vi "Last element.vi"(11 "Circuit cluster":T1) -> (3 "Last element?":bool)   [LabVIEW 2016]
uses:
  TypeDefs/Circuit Cluster.ctl
  Classes/GateAbst/GateAbst.lvclass
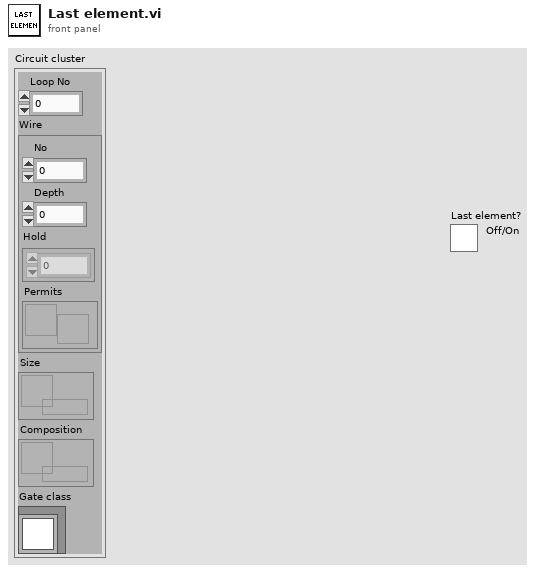
[diagram p1: front panel]
types:
  T1 = typedef "Circuit Cluster.ctl" = cluster{"Loop No":i32, "Wire":cluster{"No":i32, "Depth":i32, "Hold":i32[][], "Permits":refnum<notifier>}, "Size":refnum<queue>, "Composition":refnum<queue>, "Gate class":refnum<class "GateAbst.lvclass">}
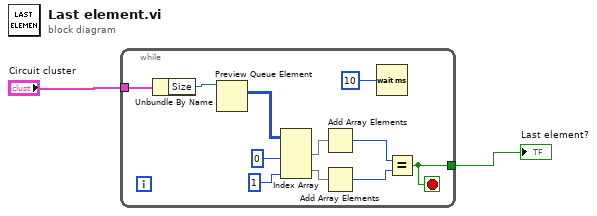
[diagram p0: block diagram]
diagram:
  n1 = while {
    tunnel: "Circuit cluster" -> [w12]
    tunnel: [w3] -> w2
    stop <- w3 stop-if-true
    n2 = Unbundle By Name(w12) -> ("Size"=w11:refnum<queue>)
    n3 = Preview Queue Element(queue=w11) -> (element=w13:i32[][])  [unwired: 2 in, 3 out]
    n4 = Index Array(array=w13, index (col) #1=0 ("disabled index (col)"), index (col) #2=1 ("index (col)")) -> (element #1=w7:i32[], element #2=w6:i32[])  [unwired: 2 in]
    n5 = Add Array Elements(numeric array=w7) -> (sum=w5:i32)
    n6 = Add Array Elements(numeric array=w6) -> (sum=w4:i32)
    n7 = Wait (ms)(milliseconds to wait=u32 10) -> ()  [unwired: 1 out]
    n8 = Equal?(x=w5, y=w4) -> (x = y?=w3:bool)
  }
  "Last element?" <- w2
